vi "Convert Variant To Boolean Array.vi"(10 "error in (no error)":errorcluster, 11 "Variant":variant) -> (2 "error out":errorcluster, 3 "Booleans":bool[](array[boolean]))   [LabVIEW 2020]
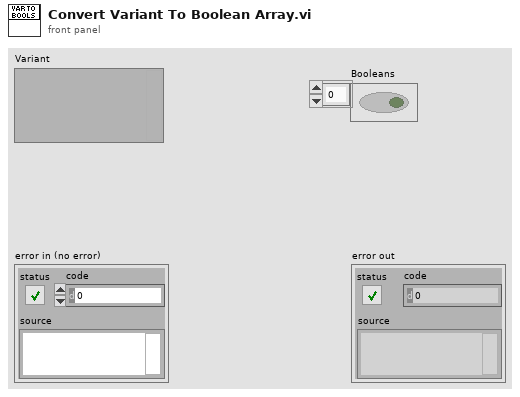
[diagram p1: front panel]
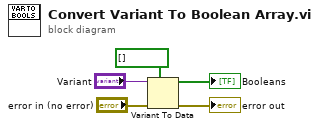
[diagram p0: block diagram]
diagram:
  n1 = Variant To Data(error in="error in (no error)", type=bool[] [], Variant="Variant") -> (data=→"Booleans":bool[], error out=→"error out":errorcluster)
